vi "_CreateDVR.vi"(10 "PrivateDataDvr":T1) -> (2 "PrivateDataDvr out":T1)   [LabVIEW 2009, in "Baby.lvclass"]
doc: "Creates a DVR for the private data cluster if it has not already been created."
uses:
  Baby.lvclass
  _PrivateDataDvr.ctl
  _PrivateData.ctl
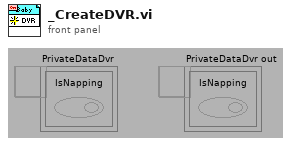
[diagram p1: front panel]
types:
  T1 = typedef "Baby.lvclass/_PrivateDataDvr.ctl" = refnum<data-value>
  T2 = typedef "Baby.lvclass/_PrivateData.ctl" = cluster{"IsNapping":bool}
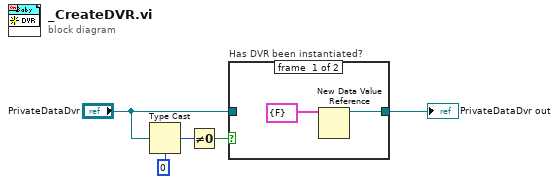
[diagram p0: block diagram]
diagram:
  n1 = Type Cast(type=0, x="PrivateDataDvr") -> (*(type *) &x=w3:i32)
  n2 = Not Equal To 0?(x=w3) -> (x != 0?=w4:bool)
  n3 = case "Has DVR been instantiated?" shown="False" w4 {
    tunnel: "PrivateDataDvr" -> [_ w8]
    tunnel: [w6 w8] -> w1
    frame #0 {
      n4 = New Data Value Reference(data value=T2 {"IsNapping"=FALSE} ("Private Data")) -> (data value reference=w6:refnum<data-value>)  [unwired: 1 in, 1 out]
    }
    frame #1 {
    }
  }
  "PrivateDataDvr out" <- w1
